vi "Get Plot at Mouse Click [AAC].vi"(8 "error in (no error)":errorcluster, 10 "Mouse Click Coordinates":T1={"Horizontal"=2147483647, "Vertical"=2147483647}, 11 "XY Graph in":T2) -> (0 "error out":errorcluster, 1 "Click is in Legend?":bool, 2 "Plot at Coordinates":i32, 3 "XY Graph out":T2, 4 "Plot Name":string, 5 "Graph Name":string, 6 "Found?":bool)   [LabVIEW 2021, in "Graphs.lvlib"]
doc: "Finds plot index at mouse click location in the specified XY Graph.\nIf not Mouse Click Coordinates are provided, returns -1 as the index, which is generally interpreted as referring to the last plot in a Graph (but not always).\n\nIf Mouse Coordinates = [I32_max,I32_max], the last plot is returned (-1 is none exist)"
uses:
  Graphs.lvlib
  XY Graph/XY Graph Refnum.ctl
  <vilib>/Utility/miscctls.llb/LVPoint32TypeDef.ctl
  Get Plot at Mouse Click in Plot Area [AAC].vi
  XY Graph/XY Graph Add-Ons.lvlib
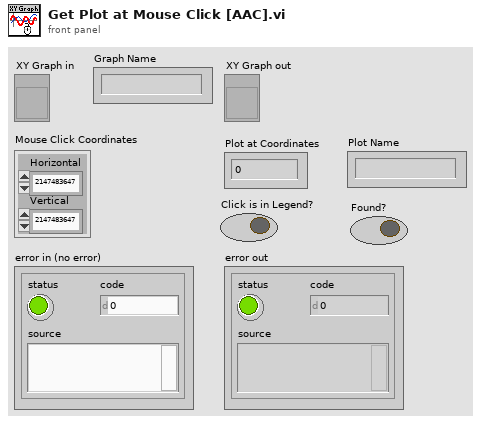
[diagram p1: front panel]
types:
  T1 = typedef "LVPoint32TypeDef.ctl" = cluster{"Horizontal":i32, "Vertical":i32}
  T2 = typedef "XY Graph Add-Ons.lvlib/XY Graph Refnum.ctl" = refnum<vi>
  T3 = typedef "LVPositionTypeDef.ctl" = cluster{"Left":i32, "Top":i32}
  T4 = typedef "LVBoundsTypeDef.ctl" = cluster{"Width":u32, "Height":u32}
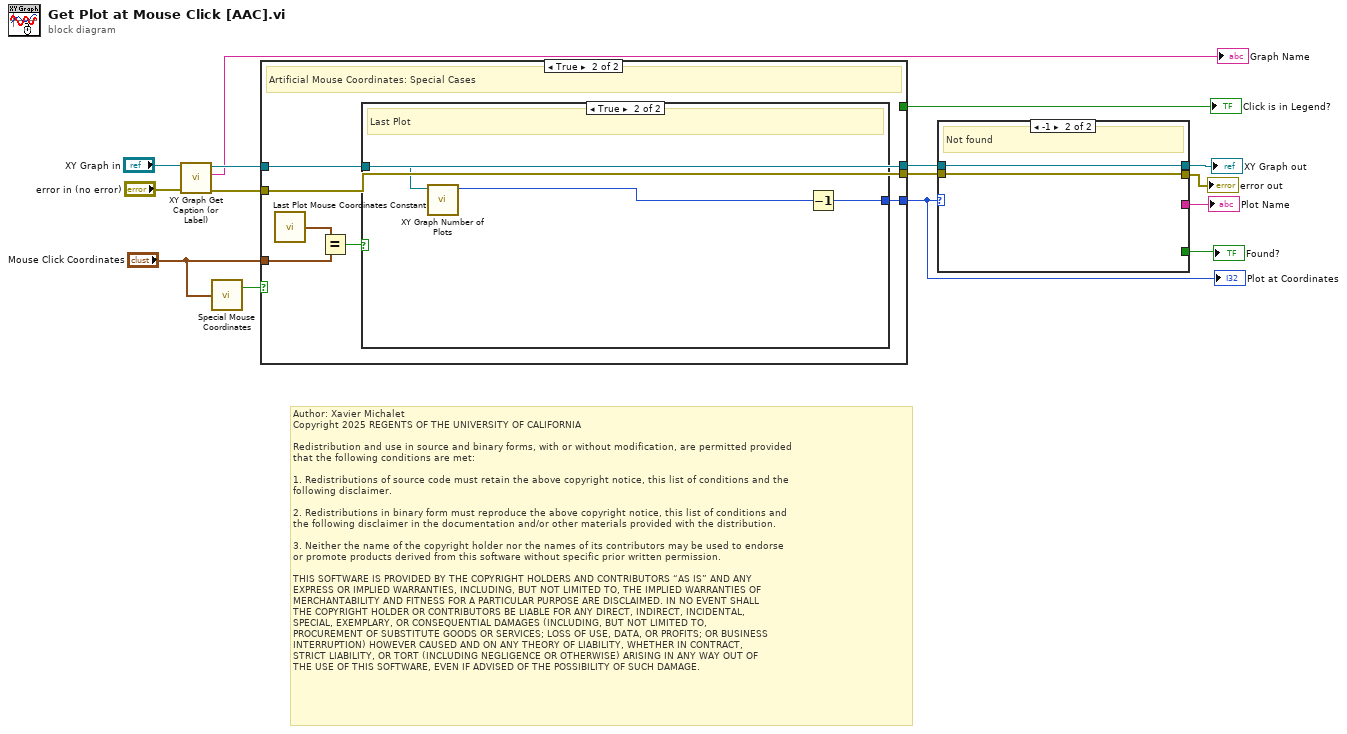
[diagram p0: block diagram]
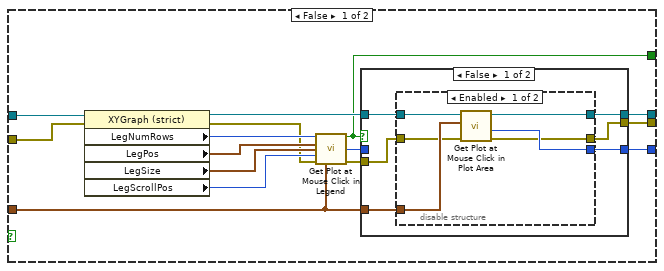
[diagram p2: hidden frame]
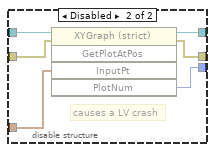
[diagram p3: hidden frame]
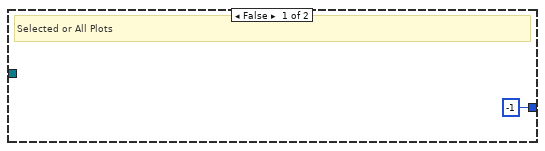
[diagram p5: hidden frame]
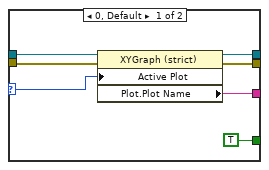
[diagram p6: hidden frame]
diagram:
  # "Author: Xavier Michalet\nCopyright 2025 REGENTS OF THE UNIVERSITY OF CALIFORNIA\n\nRedistribution and use in source and binary forms, with or without modification, are permitted provided\nthat the following conditions are met:\n\n1. Redistributions of source code must retain the above copyright notice, this list of conditions and the\nfollowing disclaimer.\n\n2. Redistributions in binary form must reproduce the above copyright notice, this list of conditions and\nthe following disclaimer in the documentation and/or other materials provided with the distribution.\n\n3. Neither the name of the copyright holder nor the names of its contributors may be used to endorse \nor promote products derived from this software without specific prior written permission.\n\nTHIS SOFTWARE IS PROVIDED BY THE COPYRIGHT HOLDERS AND CONTRIBUTORS “AS IS” AND ANY \nEXPRESS OR IMPLIED WARRANTIES, INCLUDING, BUT NOT LIMITED TO, THE IMPLIED WARRANTIES OF\nMERCHANTABILITY AND FITNESS FOR A PARTICULAR PURPOSE ARE DISCLAIMED. IN NO EVENT SHALL\nTHE COPYRIGHT HOLDER OR CONTRIBUTORS BE LIABLE FOR ANY DIRECT, INDIRECT, INCIDENTAL, \nSPECIAL, EXEMPLARY, OR CONSEQUENTIAL DAMAGES (INCLUDING, BUT NOT LIMITED TO, \nPROCUREMENT OF SUBSTITUTE GOODS OR SERVICES; LOSS OF USE, DATA, OR PROFITS; OR BUSINESS\nINTERRUPTION) HOWEVER CAUSED AND ON ANY THEORY OF LIABILITY, WHETHER IN CONTRACT, \nSTRICT LIABILITY, OR TORT (INCLUDING NEGLIGENCE OR OTHERWISE) ARISING IN ANY WAY OUT OF\nTHE USE OF THIS SOFTWARE, EVEN IF ADVISED OF THE POSSIBILITY OF SUCH DAMAGE."
  n1 = call "XY Graph Get Caption (or Label).vi"("error in (no error)"="error in (no error)", "XY Graph in"="XY Graph in") -> ("error out"=w5:errorcluster, "Caption (or Label) Text"=→"Graph Name":string, "XY Graph out"=w4:T2)  [unwired: 7 in]
  n2 = call "Special Mouse Coordinates.vi"("Mouse Click Coordinates"="Mouse Click Coordinates") -> ("Special Case (Last, Selected, All)"=w1:bool)  [unwired: 1 out]
  n3 = case shown="True" w1 {
    tunnel: [w30 w56] -> w15
    tunnel: [w27 _] -> w14
    tunnel: [w20 w55] -> w12
    tunnel: [w19 w57] -> w10
    tunnel: w5 -> [w18 w55]
    tunnel: w4 -> [w17 w56]
    tunnel: "Mouse Click Coordinates" -> [w16 w54]
    frame False {
      n4 = property class="XYGraph (strict)"(reference=w17, error in=w18) -> (reference out=w28:T2, error out=w22:errorcluster, "LegNumRows"=w29:u32, "LegPos"=w26:T3, "LegSize"=w25:T4, "LegScrollPos"=w24:u32)
      n5 = call "Get Plot at Mouse Click in Legend.vi"("LegNumRows"=w29, "Legend:Position"=w26, "Legend:Size"=w25, "LegScrollPos"=w24, "Error In"=w22, "Mouse Click Coordinates"=w16) -> ("Click is in Legend?"=w27:bool, "Plot Index"=w23:i32, "Error Out"=w21:errorcluster)  [unwired: 7 in]
      n6 = case shown="False" w27 {
        tunnel: w28 -> [w33 w51]
        tunnel: [w36 w51] -> w30
        tunnel: w23 -> [_ w50]
        tunnel: [w35 w50] -> w19
        tunnel: w16 -> [w34 _]
        tunnel: w21 -> [w32 w49]
        tunnel: [w31 w49] -> w20
        frame False {
          n7 = disable-structure shown="Enabled" {
            disable-tunnel: [w42 w47] -> w36
            disable-tunnel: [w41 w43] -> w35
            disable-tunnel: w34 -> [w40 w45]
            disable-tunnel: w33 -> [w39 w48]
            disable-tunnel: w32 -> [w38 w46]
            disable-tunnel: [w37 w44] -> w31
            frame Enabled {
              n8 = call-poly "Get Plot at Mouse Click in Plot Area.vi"("error in (no error)"=w38, "Mouse Click Coordinates (defaut: last plot)"=w40, "XYGraph Ref"=w39) -> ("error out"=w37:errorcluster, "Plot Index"=w41:i32, "XYGraph Ref"=w42:T2)  [unwired: 6 in]
            }
            frame Disabled {
              # "causes a LV crash"
              n9 = invoke class="XYGraph (strict)" method="GetPlotAtPos"(reference=w48, error in=w46, "InputPt"=w45) -> (reference out=w47:T2, error out=w44:errorcluster, "PlotNum"=w43:i32)  [unwired: 2 in, 2 out]
            }
          }
        }
        frame True {
          # "In the Legend Region"
        }
      }
    }
    frame True {
      # "Artificial Mouse Coordinates: Special Cases"
      n10 = call "Last Plot Mouse Coordinates Constant.vi"() -> ("Selected Plots Mouse Coordinates Equivalent"=w53:T1)
      n11 = Equal?(x=w53, y=w54) -> (x = y?=w52:bool)
      n12 = case shown="True" w52 {
        tunnel: [-1 w60] -> w57
        tunnel: w56 -> [_ w59]
        frame False {
          # "Selected or All Plots"
        }
        frame True {
          # "Last Plot"
          n13 = call "XY Graph Number of Plots.vi"("XYGraph in"=w59) -> ("# Plots"=w61:i32)  [unwired: 9 in, 1 out]
          n14 = Decrement(x=w61) -> (x-1=w60:i32)
        }
      }
    }
  }
  "Plot at Coordinates" <- w10
  "Click is in Legend?" <- w14
  n15 = case shown="-1" w10 {
    selector: w10 -> [w64 _]
    tunnel: w15 -> [w68 w70]
    tunnel: [w67 w70] -> w13
    tunnel: w12 -> [w66 w69]
    tunnel: [w65 w69] -> w11
    tunnel: [w63 _] -> w9
    tunnel: [TRUE ("Found?") _] -> w8
    frame 0, Default {
      n16 = property class="XYGraph (strict)"(reference=w68, error in=w66, "Active Plot"=w64) -> (reference out=w67:T2, error out=w65:errorcluster, "Plot.Plot Name"=w63:string)
    }
    frame -1 {
      # "Not found"
    }
  }
  "error out" <- w11
  "XY Graph out" <- w13
  "Plot Name" <- w9
  "Found?" <- w8
